vi "LDT Wait for Stopped then Send.vi"(7 "add to q":bool, 8 "error in (no error)":errorcluster, 9 "XML Status":string="<tcsTCSStatus>\n  <tcsVersion>V1.8</tcsVersion>\n  <accessMode>Operator</accessMode>\n  <azCurrentWrap>-1</azCurrentWrap>\n  <heartbeat>2081334</heartbeat>\n  <inPositionIsTrue>true</inPositionIsTrue>\n  <m1CoverState>Closed</m1CoverState>\n  <mountGuideMode>OpenLoop</mountGuideMode>\n  <rotCurrentWrap>-1</rotCurrentWrap>\n  <tcsHealth>WARNING</tcsHealth>\n  <tcsState>ENABLED</tcsState>\n  <currentTimes>\n    <lst>\n      <hours>12</hours>\n      <minutesTime>55</minutesTime>\n      <secondsTime>41</secondsTime>\n    </lst>\n    <time>2020-09-14T20:44:15.228+00:00</time>\n  </currentTimes>\n  <limits>\n    <moonProximity>\n      <distance_deg>51.647106572866</distance_deg>\n      <proximityFlag>false</proximityFlag>\n    </moonProximity>\n    <sunProximity>\n      <distance_deg>16.531164188648</distance_deg>\n      <proximityFlag>false</proximityFlag>\n    </sunProximity>\n    <zenith>\n      <currentZD_deg>46.221286</currentZD_deg>\n      <elZenithLimit_deg>89.3</elZenithLimit_deg>\n      <inBlindSpotIsTrue>false</inBlindSpotIsTrue>\n      <timeToBlindSpot_min>-1</timeToBlindSpot_min>\n      <timeToBlindSpotExit_min>-1</timeToBlindSpotExit_min>\n    </zenith>\n    <airmass>1.4438282807451</airmass>\n    <currentTimeToObservable_min>-1</currentTimeToObservable_min>\n    <currentTimeToUnobservable_min>262</currentTimeToUnobservable_min>\n    <timeToRotLimit_min>-1</timeToRotLimit_min>\n    <timeToAzLimit_min>-1</timeToAzLimit_min>\n  </limits>\n  <pointingPositions>\n    <azElError>\n      <azError>-0.9792</azError>\n      <elError>0.1584</elError>\n    </azElError>\n    <currentAzEl>\n      <azimuth>\n        <degreesArc>194</degreesArc>\n        <minutesArc>45</minutesArc>\n        <secondsArc>0.7</secondsArc>\n      </azimuth>\n      <elevation>\n        <degreesAlt>43</degreesAlt>\n        <minutesArc>46</minutesArc>\n        <secondsArc>43.4</secondsArc>\n      </elevation>\n    </currentAzEl>\n    <currentHA>\n      <hours>0</hours>\n      <minutesTime>44</minutesTime>\n      <secondsTime>2.04</secondsTime>\n    </currentHA>\n    <currentRADec>\n      <declination>\n        <degreesDec>-10</degreesDec>\n        <minutesArc>15</minutesArc>\n        <secondsArc>25</secondsArc>\n      </declination>\n      <equinoxPrefix>J</equinoxPrefix>\n      <equinoxYear>2000</equinoxYear>\n      <frame>FK5</frame>\n      <ra>\n        <hours>12</hours>\n        <minutesTime>10</minutesTime>\n        <secondsTime>35.34</secondsTime>\n      </ra>\n    </currentRADec>\n    <currentParAngle>12.557342470137</currentParAngle>\n    <currentRotatorPositions>\n      <rotPA>342.260103</rotPA>\n      <iaa>185.2</iaa>\n      <rotIPA>0</rotIPA>\n    </currentRotatorPositions>\n    <difftrackStatus>\n      <dAz_ArcsPS>0</dAz_ArcsPS>\n      <dEl_ArcsPS>0</dEl_ArcsPS>\n      <dRA_ArcsPS>0</dRA_ArcsPS>\n      <dDec_ArcsPS>0</dDec_ArcsPS>\n    </difftrackStatus>\n    <objectPA>\n      <EqPA>-0</EqPA>\n      <AzPA>12.557342470137</AzPA>\n    </objectPA>\n    <demandAzEl>\n      <azimuth>\n        <degreesArc>194</degreesArc>\n        <minutesArc>45</minutesArc>\n        <secondsArc>3.68</secondsArc>\n      </azimuth>\n      <elevation>\n        <degreesAlt>43</degreesAlt>\n        <minutesArc>46</minutesArc>\n        <secondsArc>42.89</secondsArc>\n      </elevation>\n    </demandAzEl>\n    <demandRADec>\n      <declination>\n        <degreesDec>-10</degreesDec>\n        <minutesArc>15</minutesArc>\n        <secondsArc>25</secondsArc>\n      </declination>\n      <equinoxPrefix>J</equinoxPrefix>\n      <equinoxYear>2000</equinoxYear>\n      <frame>FK5</frame>\n      <ra>\n        <hours>12</hours>\n        <minutesTime>10</minutesTime>\n        <secondsTime>35.24</secondsTime>\n      </ra>\n    </demandRADec>\n    <demandRotatorPositions>\n      <rotPA>342.259442</rotPA>\n    </demandRotatorPositions>\n    <targetName>unspecified</targetName>\n  </pointingPositions>\n  <OffsetStatus>\n    <offsetType>SIMPLE</offsetType>\n    <userOff1>0</userOff1>\n    <userOff2>0</userOff2>\n    <handsetOff1>0</handsetOff1>\n    <handsetOff2>0</handsetOff2>\n  </OffsetStatus>\n  <axesTrackMode>All</axesTrackMode>\n  <inPositionAzIsTrue>true</inPositionAzIsTrue>\n  <inPositionElIsTrue>true</inPositionElIsTrue>\n  <inPositionRotIsTrue>true</inPositionRotIsTrue>\n  <externalTargetCfgCmdPreviewIsTrue>true</externalTargetCfgCmdPreviewIsTrue>\n</tcsTCSStatus>", 10 "ActiveMQBroker in":refnum<class "ActiveMQBroker.lvclass">, 11 "msg to send":string) -> (0 "error out":errorcluster)   [LabVIEW 2024, in "LDT Telescope.lvclass"]
uses:
  LDT Telescope.lvclass
  TCS/DCT-related/Common/Communication/ActiveMQ/ActiveMQBroker/ActiveMQBroker.lvclass
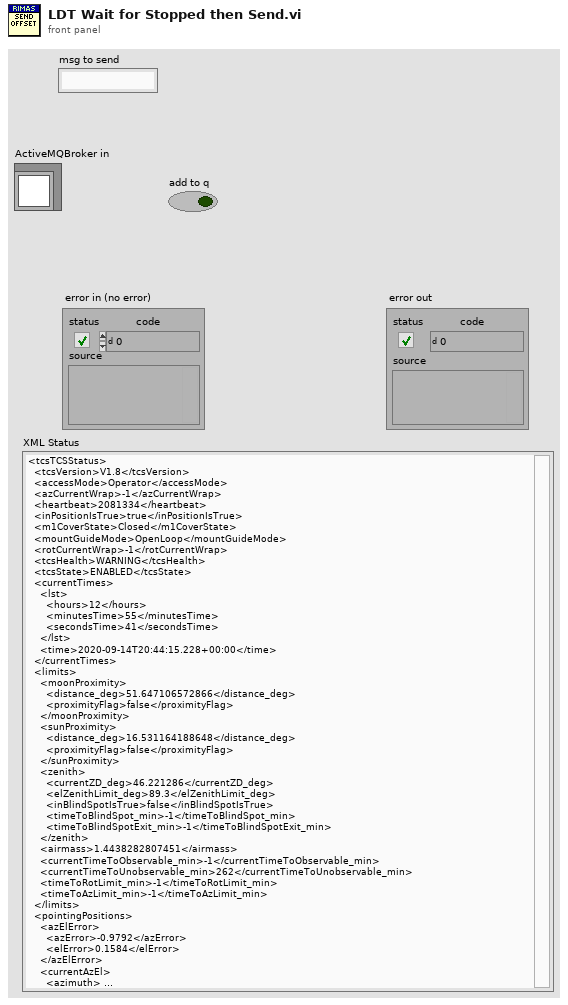
[diagram p1: front panel]
types:
  T1 = cluster{"msg":string, "timestamp":timestamp, "moved":bool}
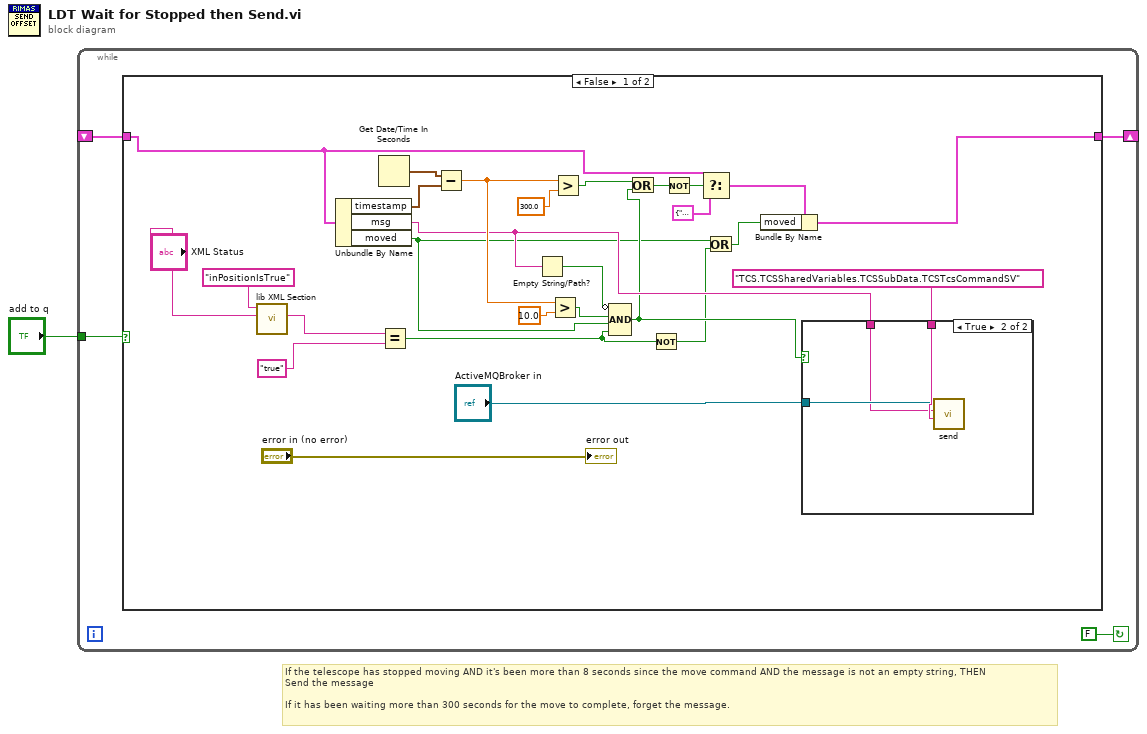
[diagram p0: block diagram]
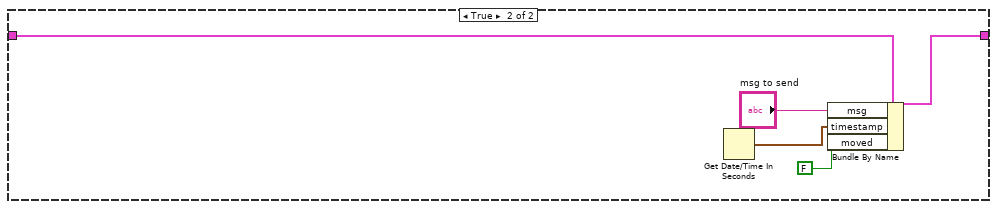
[diagram p3: hidden frame]
diagram:
  # "If the telescope has stopped moving AND it's been more than 8 seconds since the move command AND the message is not an empty string, THEN\nSend the message\n\nIf it has been waiting more than 300 seconds for the move to complete, forget the message."
  n1 = while {
    shift-right: [w5] -> _
    shift-left: _ -> [w4]
    tunnel: "add to q" -> [w2]
    stop <- FALSE continue-if-true
    n2 = case shown="False" w2 {
      tunnel: [w10 w38] -> w5
      tunnel: w4 -> [w16 w40]
      frame False {
        n3 = call "lib XML Section.vi"("XML String"="XML Status", "XML Topic"="inPositionIsTrue") -> ("XML Topic Body"=w12:string)  [unwired: 6 in, 3 out]
        n4 = Unbundle By Name(w16) -> ("timestamp"=w30:timestamp, "msg"=w23:string, "moved"=w9:bool)
        n5 = Get Date/Time In Seconds() -> (seconds since 1Jan1904=w31:timestamp)
        n6 = Equal?(x=w12, y="true") -> (x = y?=w8:bool)
        n7 = Subtract(x=w31, y=w30) -> (x-y=w27:dbl)
        n8 = Empty String/Path?(string/path=w23) -> (empty?=w22:bool)
        n9 = Greater?(x=w27, y=10.0) -> (0:w26:bool)
        n10 = Greater?(x=w27, y=300.0) -> (0:w21:bool)
        n11 = Compound Arithmetic op=AND(invert w22, w26, w9, w8) -> (w20:bool)
        n12 = Or(x=w21, y=w20) -> (x .or. y?=w19:bool)
        n13 = Not(x=w8) -> (.not. x?=w7:bool)
        n14 = Not(x=w19) -> (.not. x?=w18:bool)
        n15 = Select(t=w16, s=w18, f=T1 {"msg"="", "timestamp"=timestamp(0 s since 1904-01-01), "moved"=FALSE}) -> (s? t:f=w11:T1)
        n16 = Or(x=w9, y=w7) -> (x .or. y?=w6:bool)
        n17 = Bundle By Name(cluster=w11, "moved"=w6) -> (w10:T1)
        n18 = case shown="True" w20 {
          tunnel: "TCS.TCSSharedVariables.TCSSubData.TCSTcsCommandSV" ("topic") -> [_ w35]
          tunnel: "ActiveMQBroker in" -> [_ w34]
          tunnel: w23 -> [_ w33]
          frame False {
          }
          frame True {
            n19 = call-dynamic "send.vi"("topic"=w35, "message"=w33, "ActiveMQBroker in"=w34) -> ()  [unwired: 7 in, 2 out]
          }
        }
        "error out" <- "error in (no error)"
      }
      frame True {
        n20 = Get Date/Time In Seconds() -> (seconds since 1Jan1904=w37:timestamp)
        n21 = Bundle By Name(cluster=w40, "msg"="msg to send", "timestamp"=w37, "moved"=FALSE ("in pos")) -> (w38:T1)
      }
    }
  }
